vi "Restore File Permissions.vi"(8 "error in":errorcluster) -> (0 "error out":errorcluster)   [LabVIEW 2015]
panel:
  out "permissions":i16
  out "path out":path
  in  "path":path=path "C:/Program Files (x86)/National Instruments/RT Images/User Components"
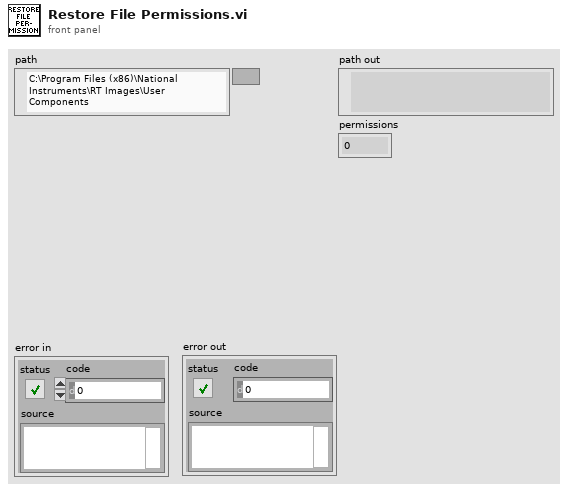
[diagram p1: front panel]
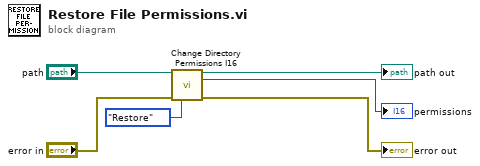
[diagram p0: block diagram]
diagram:
  n1 = call "Change Directory Permissions I16.vi"("path"="path", "error in"="error in", "Action (Get)"=enum16{"Get", "Scan", "Set", "Restore"}."Restore") -> ("path out"=→"path out":path, "permissions"=→"permissions":i16, "error out"=→"error out":errorcluster)  [unwired: 10 in]
